vi "Ramp.vi"(6 "Cycle Period":dbl, 7 "Time to Complete":dbl, 8 "error in (no error)":errorcluster, 9 "Current":dbl, 10 "End":dbl, 11 "Start":dbl) -> (0 "error out":errorcluster, 2 "New Current":dbl)   [LabVIEW 2018, in "Support Library.lvlib"]
uses:
  Support Library.lvlib
panel:
  out "Number of loops":dbl
  out "Step size":dbl
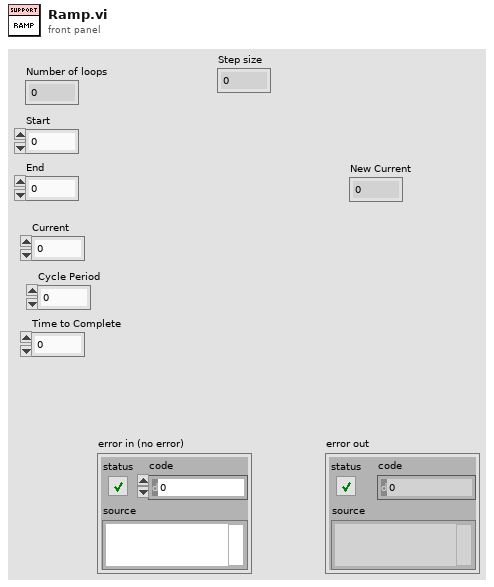
[diagram p1: front panel]
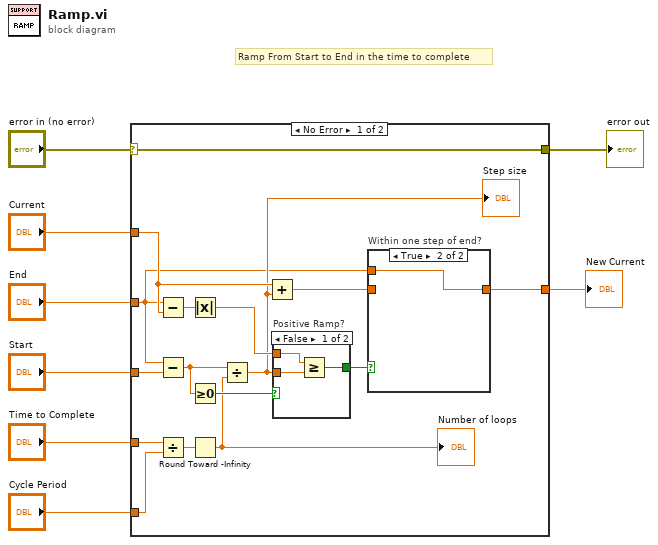
[diagram p0: block diagram]
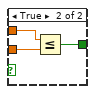
[diagram p2: hidden frame]
diagram:
  # "Ramp From Start to End in the time to complete"
  n1 = case shown="No Error" "error in (no error)" {
    selector: "error in (no error)" -> [w24 w33]
    tunnel: [w24 w33] -> w2
    tunnel: "Start" -> [w13 _]
    tunnel: "End" -> [w14 _]
    tunnel: "Time to Complete" -> [w23 _]
    tunnel: "Cycle Period" -> [w22 _]
    tunnel: "Current" -> [w20 w34]
    tunnel: [w16 w34] -> w3
    frame No Error {
      n2 = Subtract(x=w14, y=w20) -> (x-y=w21:dbl)
      n3 = Subtract(x=w14, y=w13) -> (x-y=w12:dbl)
      n4 = Divide(x=w23, y=w22) -> (x/y=w10:dbl)
      n5 = Absolute Value(x=w21) -> (abs(x)=w19:dbl)
      n6 = Greater Or Equal To 0?(x=w12) -> (x >= 0?=w11:bool)
      n7 = Round Toward -Infinity(1:w10) -> (0:w9:dbl)
      "Number of loops" <- w9
      n8 = Divide(x=w12, y=w9) -> (x/y=w18:dbl)
      "Step size" <- w18
      n9 = Add(x=w20, y=w18) -> (x+y=w15:dbl)
      n10 = case "Positive Ramp?" shown="False" w11 {
        tunnel: w19 -> [w26 w30]
        tunnel: w18 -> [w27 w29]
        tunnel: [w25 w28] -> w17
        frame False {
          n11 = Greater Or Equal?(x=w26, y=w27) -> (x >= y?=w25:bool)
        }
        frame True {
          n12 = Less Or Equal?(x=w30, y=w29) -> (x <= y?=w28:bool)
        }
      }
      n13 = case "Within one step of end?" shown="True" w17 {
        tunnel: [w31 w32] -> w16
        tunnel: w14 -> [_ w32]
        tunnel: w15 -> [w31 _]
        frame False {
        }
        frame True {
        }
      }
    }
    frame Error {
    }
  }
  "New Current" <- w3
  "error out" <- w2
